vi "AOD Control - debugging(host).vi"() -> ()   [LabVIEW 2012]
uses:
  <vilib>/rvi/interface/nirviOpenFPGA/nirviOpenFPGA.xnode
  <vilib>/rvi/interface/nirviReadWriteControl/nirviReadWriteControl.xnode
  <vilib>/userdefined/High Color/nirio_resource_hc.ctl
  <vilib>/rvi/interface/nirviMethod/nirviMethod.xnode
  FPGA Bitfiles/AOD Control.lvproj_FPGA Target_AOD Control (FPGA)~D2.lvbitx
  AOD Control (FPGA).vi
  <vilib>/Waveform/DWDTOps.llb/DWDT Binary U16 to Digital.vi
  <vilib>/rvi/interface/RandomDataEmulation/nirviRandomDataOpen.vi
  <vilib>/rvi/errors/niLvFpgaMergeErrorWithErrorCode.vi
panel:
  in  "TriggerAcq":bool=TRUE
  out "State":T1(ring)
  out "SerialError":bool
  in  "Abort":bool
  out "Acquire":bool
  out "SampleCount":i16
  in  "AcqDivider":i32=10
  in  "Downsample":i32=160
  in  "Reset":bool
  in  "SclkDivider":u32=40
  in  "Pause":u32
  in  "P":bool
  in  "Volume Scan":bool
  in  "Scan Settings":T2={"XStart"=-200000000, "XEnd"=200000000, "XInc"=20000000, "YStart"=-200000000, "YEnd"=200000000, "YInc"=20000000, "ZStart"=-40000, "ZEnd"=40000, "ZInc"=400}
  out "PointTime":u32
  out "NumReps":i32
  out "NumPoints":i32
  out "Read Point":cluster{"X":i32, "Y":i32, "Z":i32}
  out "PointNum":u32
  out "Sequencing error":bool
  out "Count":i32
  in  "Points":i32[][](array[numeric])
  in  "Scans":i32
  in  "Scan":bool
  out "Write count":i32
  out "Written":cluster{"Address":u8, "Value":u32}[](array[cluster]) {"Address" format="%x"; "Value" format="%x"}
  in  "Write Point":bool
  in  "Write Registers":cluster{"Address":u8, "Value":u32}[](array[cluster])=[{"Address"=0, "Value"=240}, {"Address"=1, "Value"=13762592}, {"Address"=2, "Value"=32768}, {"Address"=3, "Value"=8413952}, {"Address"=4, "Value"=0}, {"Address"=5, "Value"=0}, {"Address"=6, "Value"=1023}, {"Address"=7, "Value"=257}, {"Address"=8, "Value"=21}, {"Address"=0, "Value"=246}] {"Address" format="%x"; "Value" format="%x"}
  in  "UpdatesPerPoint":u32=2000
  in  "Write Point":cluster{"X":i32, "Y":i32, "Z":i32}
  in  "Samples":u32=1000
  in  "WriteSize":enum16{"1", "2", "4"}(ring)
  in  "Loopback delay":u32=4
  out "ControlSignals":digitalwaveform(graph)
  out "Elements Remaining":u32
  in  "Stop":bool
  in  "Write Register":bool
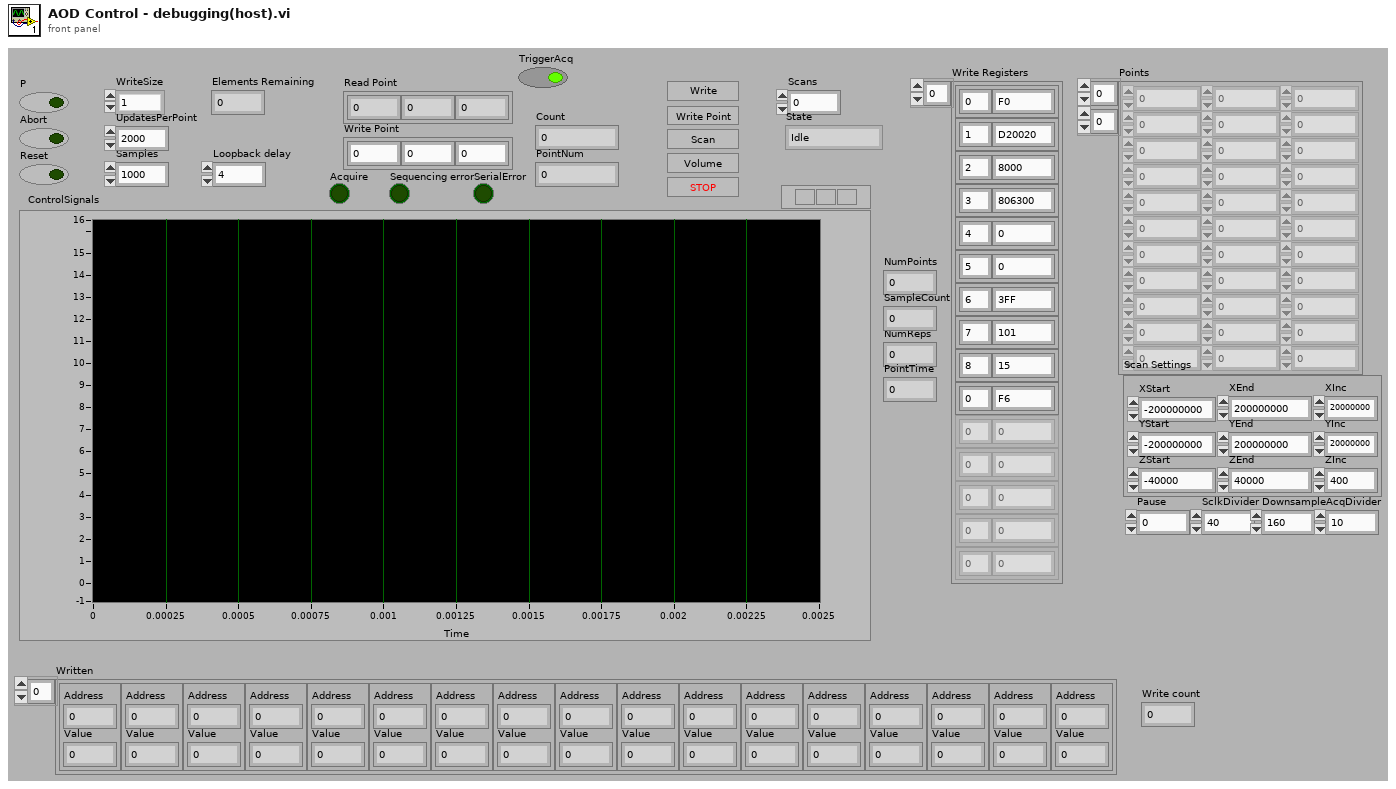
[diagram p1: front panel]
types:
  T1 = enum16{"Idle", "Write Registers", "Receive Points", "Prepare Volume", "Arm Scan", "Scan Points"}
  T2 = cluster{"XStart":i32, "XEnd":i32, "XInc":i32, "YStart":i32, "YEnd":i32, "YInc":i32, "ZStart":i32, "ZEnd":i32, "ZInc":i32}
  T3 = typedef "nirio_resource_hc.ctl" = tag
  T4 = enum16{"Idle", "Write Registers", "Receive Points", "Scan Points"}
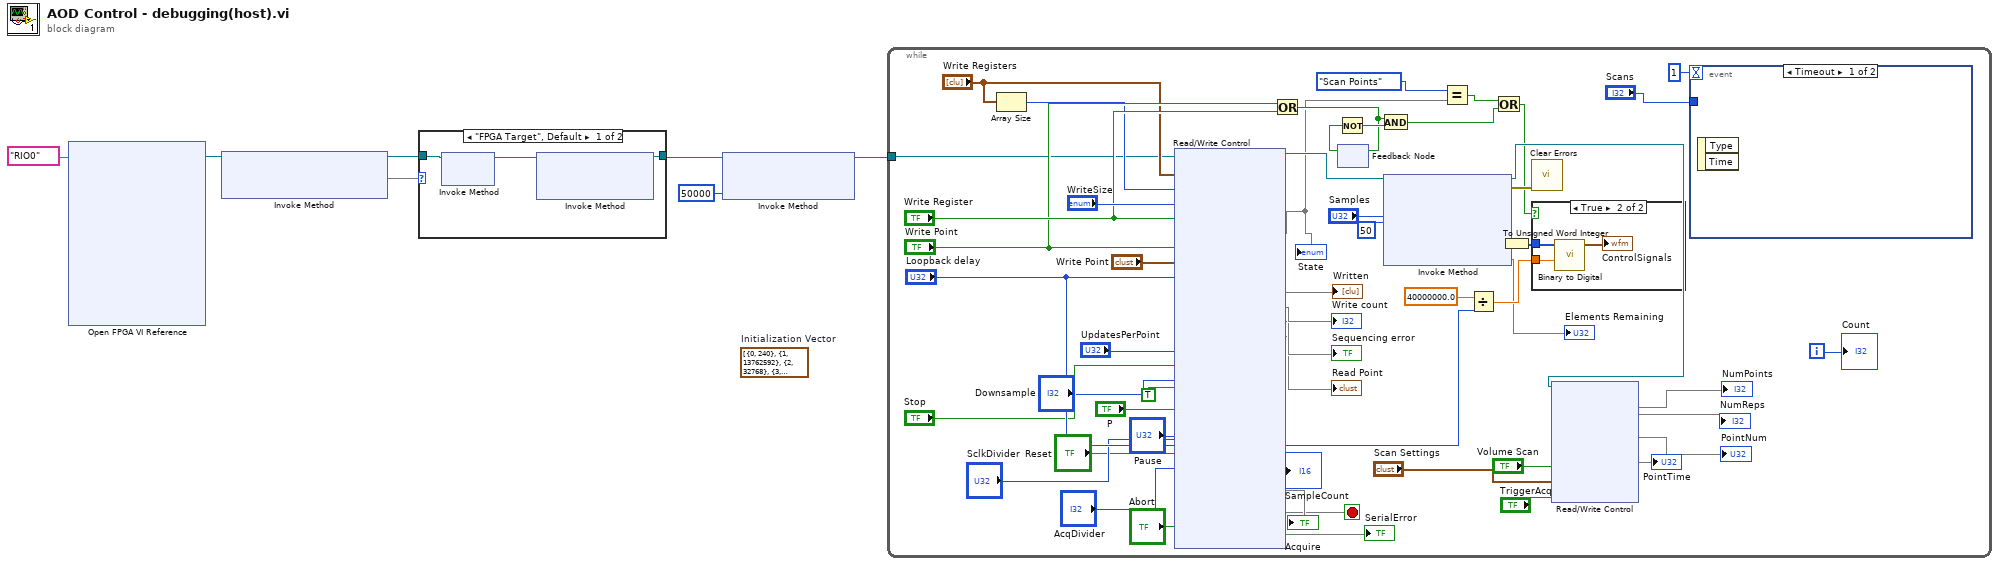
[diagram p0: block diagram]
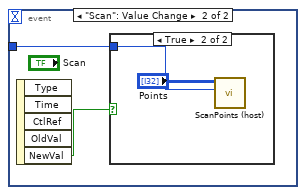
[diagram p3: hidden frame]
diagram:
  (unwired) cluster{"Address":u8, "Value":u32}[] [{"Address"=0, "Value"=240}, {"Address"=1, "Value"=13762592}, {"Address"=2, "Value"=32768}, {"Address"=3, "Value"=8413952}, {"Address"=4, "Value"=0}, {"Address"=5, "Value"=0}, {"Address"=6, "Value"=1023}, {"Address"=7, "Value"=257}, {"Address"=8, "Value"=21}, {"Address"=0, "Value"=246}]  # Initialization Vector
  n1 = xnode "Open FPGA VI Reference"("resource name"=T3 "RIO0") -> ("FPGA VI Reference Out"=w4:refnum<k20>)  [unwired: 1 in, 1 out]
  n2 = xnode "Invoke Method"("FPGA VI Reference In"=w4) -> ("FPGA VI Reference Out"=w2:refnum<k20>, "FPGA VI Execution Mode"=w3)  [unwired: 1 in, 1 out]
  n3 = case shown="\"FPGA Target\", Default" w3 {
    tunnel: [w8 w11] -> w5
    tunnel: w2 -> [w9 w11]
    frame "FPGA Target", Default {
      n4 = xnode "Invoke Method"("FPGA VI Reference In"=w9) -> ("FPGA VI Reference Out"=w10:refnum<k20>)  [unwired: 1 in, 1 out]
      n5 = xnode "Invoke Method"("FPGA VI Reference In"=w10) -> ("FPGA VI Reference Out"=w8:refnum<k20>)  [unwired: 2 in, 1 out]
    }
    frame "Development Computer with Simulated I/O" {
    }
  }
  n6 = xnode "Invoke Method"("FPGA VI Reference In"=w5, "Depth"=u32 50000) -> ("FPGA VI Reference Out"=w6:refnum<k20>)  [unwired: 1 in, 1 out]
  n7 = while {
    tunnel: w6 -> [w48]
    i -> [w47]
    stop <- w17 stop-if-true
    n8 = Array Size(array="Write Registers") -> (size(s)=w51:i32)
    n9 = xnode "Read/Write Control"("FPGA VI Reference In"=w48, "Register Writes"="Write Registers", "Number Registers"=w51, "WriteSize"="WriteSize", "Write Register"="Write Register", "Write Point"="Write Point", "Point"="Write Point", "Loopback delay"="Loopback delay", "UpdatesPerPoint"="UpdatesPerPoint", "stop"="Stop", "Downsample"="Downsample", "Loopback"=TRUE, "P"="P", "Pause"="Pause", "SclkDivider"="SclkDivider", "Reset"="Reset", "AcqDivider"="AcqDivider", "Abort"="Abort") -> ("FPGA VI Reference Out"=w57:refnum<k20>, "State"=w14, "Written"=→"Written", "Write count"=→"Write count", "Sequencing error"=→"Sequencing error", "Point"=→"Read Point", "SampleCount"=→"SampleCount", "Acquire"=→"Acquire", "Stopped"=w17, "SerialError"=→"SerialError")  [unwired: 1 in, 1 out]
    "State" <- w14
    n10 = Or(x="Write Point", y="Write Register") -> (x .or. y?=w55:bool)
    n11 = feedback-in #1(w55) -> ()
    n12 = feedback #1() -> (w59:bool)  [unwired: 1 in]
    n13 = Not(x=w59) -> (.not. x?=w58:bool)
    n14 = And(x=w55, y=w58) -> (x .and. y?=w22:bool)
    n15 = xnode "Invoke Method"("FPGA VI Reference In"=w57, "Number of Elements"="Samples", "Timeout (ms)"=50) -> ("FPGA VI Reference Out"=w37:refnum<k20>, "error out"=w64:errorcluster, "Data"=w43:void[], "Elements Remaining"=→"Elements Remaining")  [unwired: 1 in]
    n16 = Equal?(x=T4."Scan Points" ("State"), y=w14) -> (x = y?=w23:bool)
    n17 = Divide(x=40000000.0, y="Loopback delay") -> (x/y=w63:dbl)
    n18 = Or(x=w23, y=w22) -> (x .or. y?=w21:bool)
    n19 = To Unsigned Word Integer(number=w43) -> (unsigned 16bit integer=w42:u16[])
    n20 = call <vilib>:"Clear Errors.vi"("error in (no error)"=w64) -> ()  [unwired: 6 in, 1 out]
    n21 = case shown="True" w21 {
      tunnel: w42 -> [_ w71]
      tunnel: w63 -> [_ w70]
      frame False {
      }
      frame True {
        n22 = call-poly <vilib>:"Binary to Digital.vi"("sample rate"=w70, "binary array"=w71) -> ("digital waveform"=→"ControlSignals":digitalwaveform)  [unwired: 8 in, 1 out]
      }
    }
    n23 = xnode "Read/Write Control"("FPGA VI Reference In"=w37, "Volume Scan"="Volume Scan", "Scan Settings"="Scan Settings", "TriggerAcq"="TriggerAcq") -> ("NumPoints"=→"NumPoints", "NumReps"=→"NumReps", "PointNum"=→"PointNum", "PointTime"=→"PointTime")  [unwired: 1 in, 2 out]
    n24 = event shown="[0] Timeout" {
      selector: _ -> [_ _]
      dyn-events: _ -> [_ _]
      timeout: 1 -> [_ _]
      tunnel: "Scans" -> [_ w66]
      event Timeout {
        n25 = event-data() -> ()  [unwired: 1 in, 2 out]
      }
      event "Scan": Value Change {
        n26 = event-data() -> ("NewVal"=w67:bool)  [unwired: 1 in, 4 out]
        n27 = case shown="True" w67 {
          tunnel: w66 -> [_ w68]
          frame False {
          }
          frame True {
            n28 = call "ScanPoints (host).vi"("Points"=w68, "FPGA VI Reference Out"="Points") -> ()  [unwired: 10 in]
          }
        }
      }
    }
    "Count" <- w47
  }
